vi "changeLED_event.vi"(0 "eventcluster":T1, 1 "LED?":string, 5 "string?":string, 7 "newStatus":bool=TRUE, 9 "ctlarr":T2, 11 "error in (no error)":errorcluster) -> (4 "eventclusterOut":T1, 10 "ctlarrOut":T2, 15 "error out":errorcluster)   [LabVIEW 2017]
uses:
  RefArray/RefArray.ctl
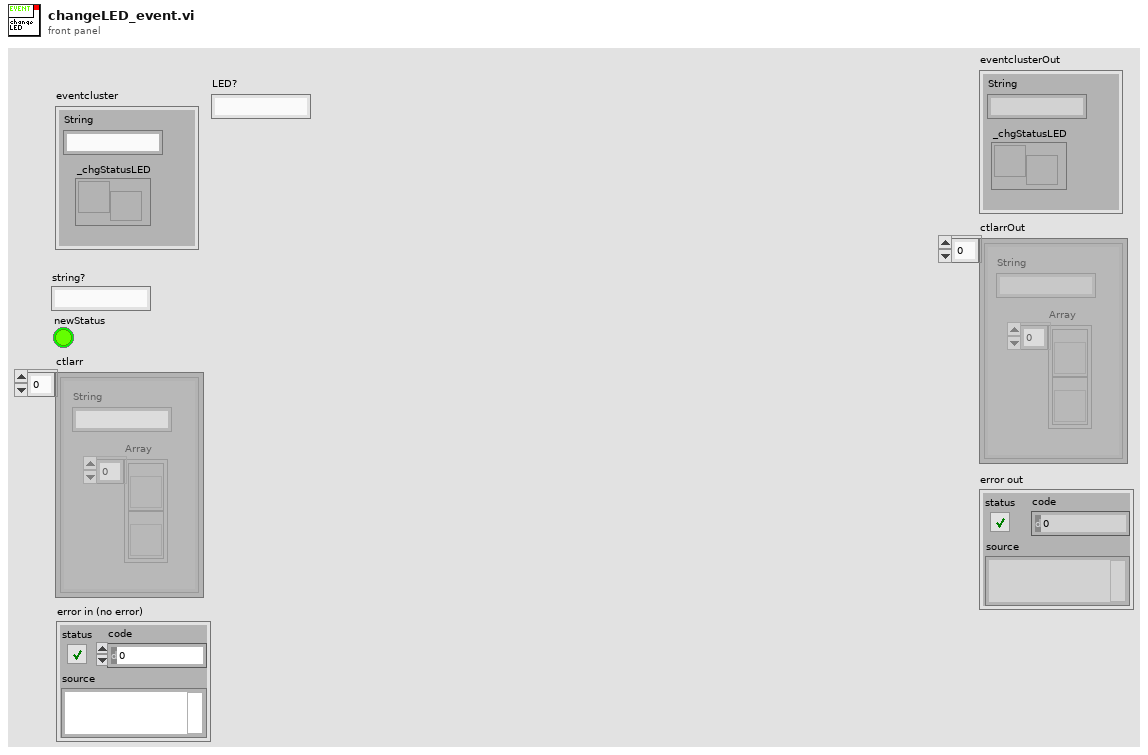
[diagram p1: front panel]
types:
  T1 = cluster{"String":string, "_chgStatusLED":refnum<user-event>}
  T2 = typedef "RefArray.ctl" = cluster{"String":string, "Array":refnum<vi>[]}[]
  T3 = cluster{"string?":string, "ctlref":refnum<vi>, "newStatus":bool, "ctlstr":refnum<vi>}
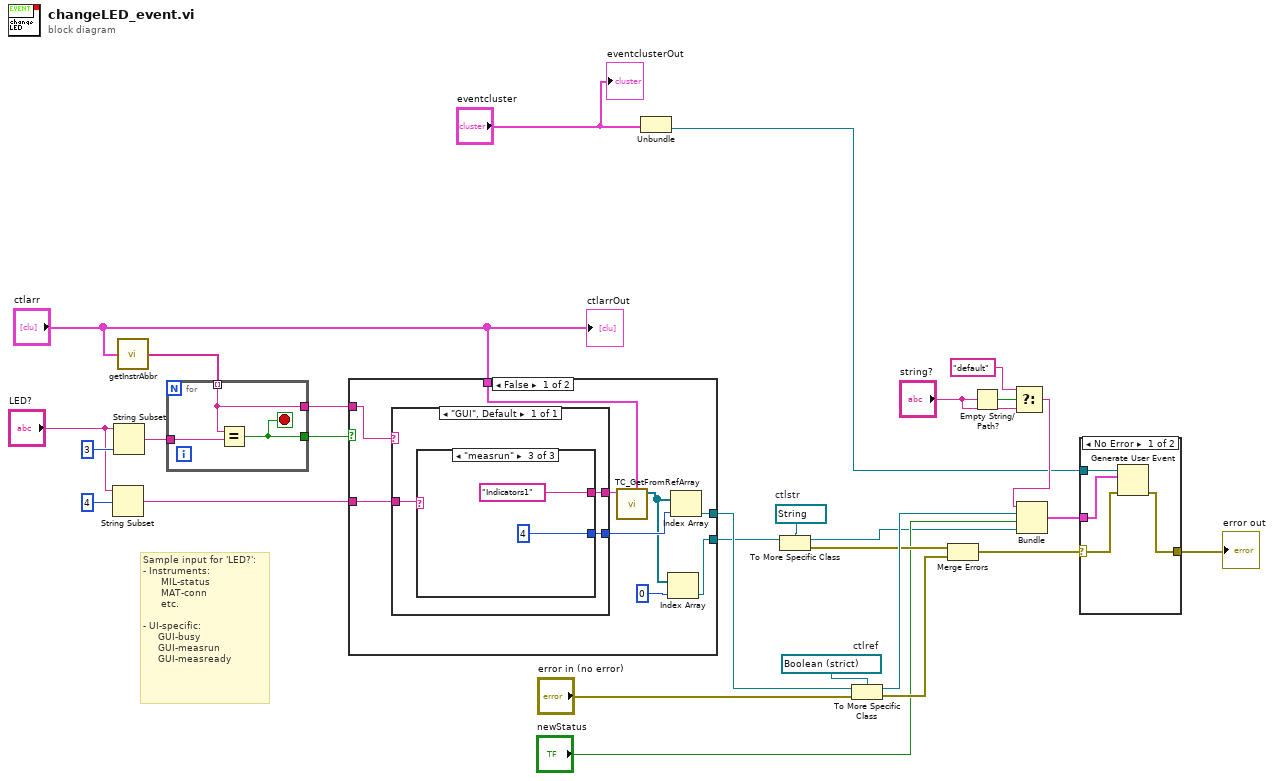
[diagram p0: block diagram]
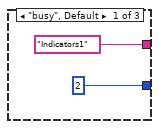
[diagram p2: hidden frame]
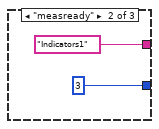
[diagram p3: hidden frame]
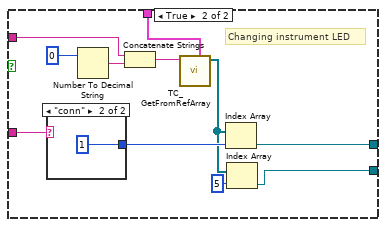
[diagram p4: hidden frame]
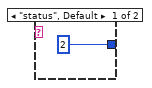
[diagram p5: hidden frame]
diagram:
  w7 = refnum<vi> refnum  # ctlstr
  w28 = refnum<vi> refnum  # ctlref
  # "Sample input for 'LED?':\n- Instruments:\n      MIL-status\n      MAT-conn\n      etc.\n\n- UI-specific:\n     GUI-busy\n     GUI-measrun\n     GUI-measready"
  n1 = String Subset(string="LED?", offset (0)=4) -> (substring=w14:string)  [unwired: 1 in]
  n2 = String Subset(string="LED?", length (rest)=3) -> (substring=w19:string)  [unwired: 1 in]
  n3 = call "getInstrAbbr.vi"("ctlarr"="ctlarr") -> ("abbrArray"=w13:string[])
  n4 = for {
    tunnel: w13 -> [w29] mode=indexing
    tunnel: w19 -> [w31]
    tunnel: [w30] -> w18
    tunnel: [w29] -> w17
    stop <- w30 stop-if-true
    n5 = Equal?(x=w29, y=w31) -> (x = y?=w30:bool)
  }
  n6 = case shown="False" w18 {
    tunnel: w17 -> [w40 w57]
    tunnel: w14 -> [w39 w55]
    tunnel: "ctlarr" -> [w37 w56]
    tunnel: [w38 w53] -> w11
    tunnel: [w33 w50] -> w1
    frame False {
      n7 = case shown="\"GUI\", Default" w40 {
        tunnel: w39 -> [w43]
        tunnel: [w42] -> w36
        tunnel: [w41] -> w35
        frame "GUI", Default {
          n8 = case shown="\"measrun\"" w43 {
            tunnel: [2 3 4] -> w42
            tunnel: ["Indicators1" "Indicators1" "Indicators1"] -> w41
            frame "busy", Default {
            }
            frame "measready" {
            }
            frame "measrun" {
            }
          }
        }
      }
      n9 = call "TC_GetFromRefArray.vi"("arrayIn"=w37, "NameToFind"=w35) -> ("refArray"=w34:refnum<vi>[])  [unwired: 8 in, 1 out]
      n10 = Index Array(array=w34, index=0) -> (element=w33:refnum<vi>)
      n11 = Index Array(array=w34, index=w36) -> (element=w38:refnum<vi>)
    }
    frame True {
      # "Changing instrument LED"
      n12 = case shown="\"conn\"" w55 {
        tunnel: [2 1] -> w54
        frame "status", Default {
        }
        frame "conn" {
        }
      }
      n13 = Number To Decimal String(number=0) -> (decimal integer string=w59:string)  [unwired: 1 in]
      n14 = Concatenate Strings(w57, w59) -> (w60:string)
      n15 = call "TC_GetFromRefArray.vi"("arrayIn"=w56, "NameToFind"=w60) -> ("refArray"=w52:refnum<vi>[])  [unwired: 8 in, 1 out]
      n16 = Index Array(array=w52, index=w54) -> (element=w53:refnum<vi>)
      n17 = Index Array(array=w52, index=5) -> (element=w50:refnum<vi>)
    }
  }
  n18 = Unbundle("eventcluster") -> ("_chgStatusLED"=w10:refnum<user-event>)  [unwired: 1 out]
  n19 = To More Specific Class(target class=w7, reference=w1) -> (specific class reference=w2:refnum<vi>, error out=w4:errorcluster)  [unwired: 1 in]
  n20 = To More Specific Class(target class=w28, reference=w11, error in="error in (no error)") -> (specific class reference=w8:refnum<vi>, error out=w5:errorcluster)
  n21 = Merge Errors(w4, w5) -> (w6:errorcluster)
  n22 = Empty String/Path?(string/path="string?") -> (empty?=w26:bool)
  n23 = Select(t="default", s=w26, f="string?") -> (s? t:f=w23:string)
  n24 = Bundle("string?"=w23, "ctlref"=w8, "newStatus"="newStatus", "ctlstr"=w2) -> (w27:T3)  [unwired: 1 in]
  n25 = case shown="No Error" w6 {
    selector: w6 -> [w64 w67]
    tunnel: w10 -> [w66 _]
    tunnel: w27 -> [w65 _]
    tunnel: [w63 w67] -> w22
    frame No Error {
      n26 = Generate User Event(user event=w66, event data cluster=w65, error in=w64) -> (error out=w63:errorcluster)  [unwired: 1 in, 1 out]
    }
    frame Error {
    }
  }
  "error out" <- w22
  "ctlarrOut" <- "ctlarr"
  "eventclusterOut" <- "eventcluster"
